vi "UDP Rx Process.vi"(10 "Parameters":variant, 11 "Process":refnum<class "Process.lvclass">) -> ()   [LabVIEW 2019, in "UDP-Custom-Device Engine.lvlib"]
uses:
  UDP-Custom-Device Engine.lvlib
  <vilib>/NI/NIVS Inline Async API/_VS Inline Async API/Process/Process.lvclass
  <vilib>/NI/NIVS Inline Async API/_VS Inline Async API/Process/Process.lvclass/Process.ctl
  <vilib>/NI/NIVS Inline Async API/_VS Inline Async API/Process/Data Member Access/Read Data Access.vi
  <vilib>/NI/NIVS Inline Async API/_VS Inline Async API/Error Handling Process/SubVIs/Error.ConvertArray.vi
  <vilib>/NI/NIVS Inline Async API/_Data Access Engine/Data Access Engine/Data Access Engine.lvclass
  <vilib>/NI VeriStand/VeriStand Data/VeriStand Data.lvlib
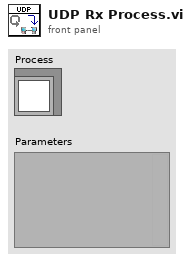
[diagram p1: front panel]
types:
  T1 = typedef "UDP-Custom-Device Engine.lvlib/Engine - Rx Loop Data.ctl" = cluster{"General Resources":T2, "Header Details":T4, "Data Conversion":T6, "Runtime Resources":T8, "New Data Support":T11, "Channel Resources":T13, "Debug Resources":T15}
  T2 = typedef "UDP-Custom-Device Engine.lvlib/Engine - General Resources.ctl" = cluster{"Packet Name":string, "Packet ID":i32, "Local IP Address":string, "Local Port":i32, "Multicast":bool, "Multicast IP Address":u32, "Header Info":bool[], "Byte Order":enum16{"big-endian, network order", "native, host order", "little-endian"}, "Channel Data Types":T3[], "Duplex Packets":refnum<data-value>}
  T3 = typedef "VeriStand Data.lvlib/Typedefs.Data Types.ctl" = enum16{"Boolean", "Single", "Double", "I8", "I16", "I32", "I64", "U8", "U16", "U32", "U64"}
  T4 = typedef "UDP-Custom-Device Shared.lvlib/Shared - Header Details.ctl" = cluster{"Packet Size":u16, "Protocol Revision":u8, "System Definition Version":u64, "Source Node Name":string, "Packet ID":u32, "Number of Channels":u32, "Static Header Size":u16, "Total Header Size":u16, "CustomHeaderLogic":T5}
  T5 = typedef "UDP-Custom-Device Shared.lvlib/Shared - Custom Header.ctl" = cluster{"CustomHeaderON":bool, "CustomHeaderLogic":string}
  T6 = typedef "UDP-Custom-Device Engine.lvlib/Engine - Data Conversion Config.ctl" = cluster{"Byte Buffer":refnum<class "Byte Buffer.lvclass">, "Data Pointers":u64[], "Channel Count":i32, "Mappings":T7[], "Static Header Payload":string, "Packet Count":dbl, "Packet Size":i32}
  T7 = typedef "VeriStand Data.lvlib/Byte Buffer.lvclass/Byte Buffer.Mapping.ctl" = cluster{"pointer":u64, "count":i64, "buffer offset":u64, "data type":T3}
  T8 = typedef "UDP-Custom-Device Engine.lvlib/Engine - Rx Runtime Resources.ctl" = cluster{"Connection ID":refnum<k16>, "Timeout":i32, "ExecutionConfig":T9}
  T9 = typedef "UDP-Custom-Device Engine.lvlib/Engine - Execution Config.ctl" = cluster{"Loop Period":i64, "RT Loop Period":i64, "Untimed Period":u32, "Target Processor":i32, "Priority":i32, "Thread Management":T10}
  T10 = typedef "UDP-Custom-Device Shared.lvlib/Shared - Thread Management.ctl" = enum16{"Untimed (Default)", "Timed (High Priority)"}
  T11 = typedef "UDP-Custom-Device Engine.lvlib/Engine - Rx New Data Options Support.ctl" = cluster{"New Data Option":T12, "Packet Count":dbl}
  T12 = typedef "UDP-Custom-Device Shared.lvlib/Shared - New Data Options.ctl" = enum16{"Timeout Reset", "Counter"}
  T13 = typedef "UDP-Custom-Device Engine.lvlib/Engine - Rx Channel Refs.ctl" = cluster{"Receive Channels":T14, "New Data":T14, "Port":T14}
  T14 = typedef "Data Access Engine.lvlib/Data Access Engine.lvclass/Write.DVR.ctl" = refnum<data-value>
  T15 = typedef "UDP-Custom-Device Engine.lvlib/Engine - Debug Resources.ctl" = cluster{"Debug Mode":bool, "Debug Log File":refnum<file>, "Packet Name":string}
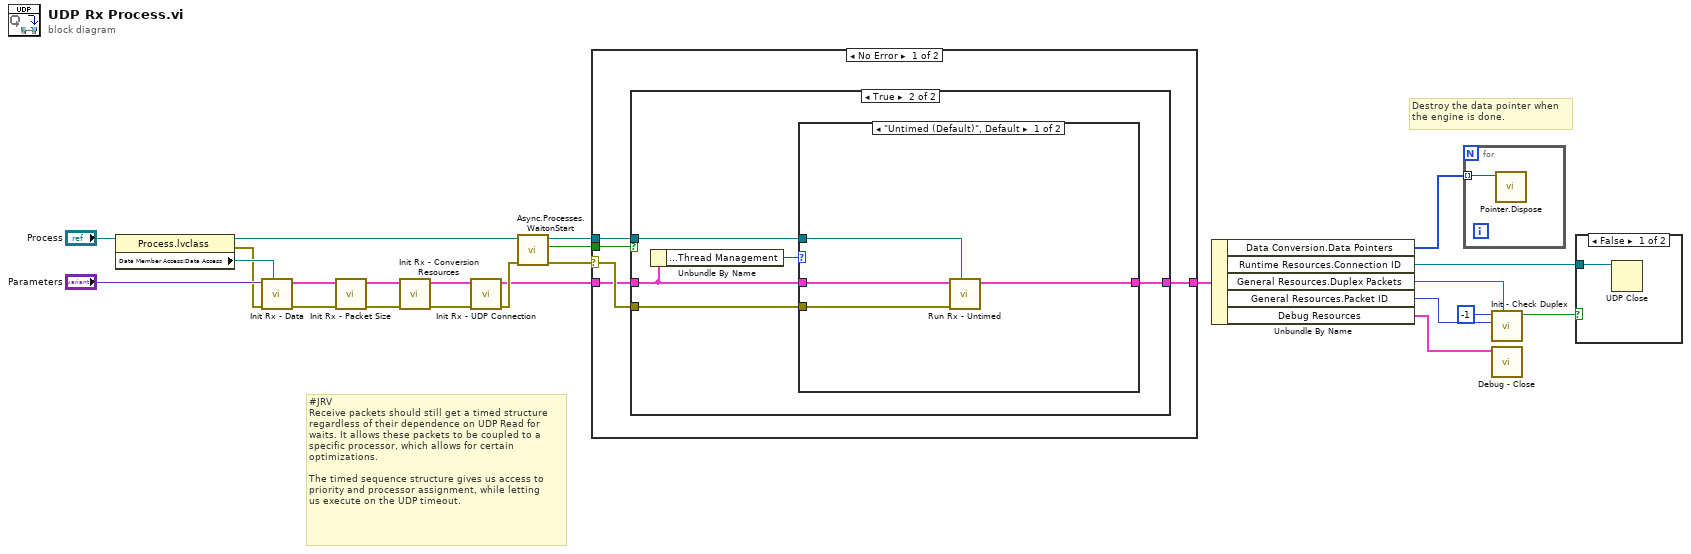
[diagram p0: block diagram]
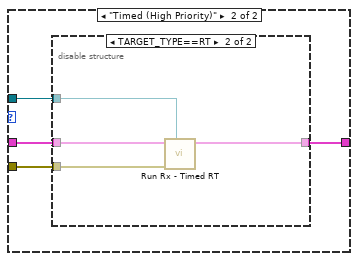
[diagram p3: hidden frame]
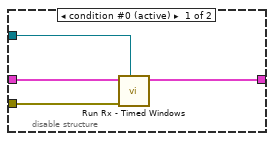
[diagram p4: hidden frame]
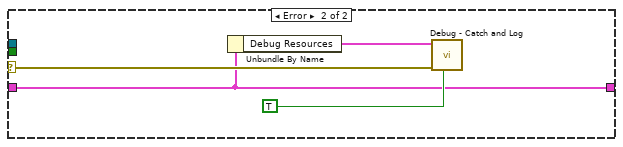
[diagram p5: hidden frame]
diagram:
  # "#JRV\nReceive packets should still get a timed structure\nregardless of their dependence on UDP Read for\nwaits. It allows these packets to be coupled to a\nspecific processor, which allows for certain \noptimizations.\n\nThe timed sequence structure gives us access to\npriority and processor assignment, while letting\nus execute on the UDP timeout."
  # "Destroy the data pointer when\nthe engine is done."
  n1 = property class="Process.lvclass"(reference="Process") -> (reference out=w24:refnum<class "Process.lvclass">, error out=w20:errorcluster, "Data Member Access:Data Access"=w21:refnum<class "Data Access Engine.lvclass">)  [unwired: 1 in]
  n2 = call "Init Rx - Data.vi"("Data Access in"=w21, "error in (no error)"=w20, "Parameters"="Parameters") -> ("error out"=w10:errorcluster, "Rx Loop Data"=w12:T1)  [unwired: 6 in, 1 out]
  n3 = call "Init Rx - Packet Size.vi"("error in (no error)"=w10, "Rx Loop Data"=w12) -> ("error out"=w9:errorcluster, "Rx Loop Data out"=w11:T1)  [unwired: 8 in]
  n4 = call "Init Rx - Conversion Resources.vi"("error in (no error)"=w9, "Rx Loop Data"=w11) -> ("error out"=w13:errorcluster, "Rx Loop Data out"=w14:T1)  [unwired: 8 in]
  n5 = call "Init Rx - UDP Connection.vi"("error in (no error)"=w13, "Rx Loop Data in"=w14) -> ("error out"=w16:errorcluster, "Rx Loop Data out"=w6:T1)  [unwired: 8 in]
  n6 = call <vilib>:"Async.Processes.WaitonStart.vi"("error in (no error)"=w16, "Process"=w24) -> ("error out"=w19:errorcluster, "Execute"=w17:bool, "Process out"=w18:refnum<class "Process.lvclass">)  [unwired: 7 in]
  n7 = case shown="No Error" w19 {
    selector: w19 -> [w27 w53]
    tunnel: w17 -> [w29 _]
    tunnel: w18 -> [w28 _]
    tunnel: w6 -> [w26 w52]
    tunnel: [w25 w52] -> w15
    frame No Error {
      n8 = case shown="True" w29 {
        tunnel: w27 -> [_ w34]
        tunnel: w28 -> [_ w35]
        tunnel: w26 -> [w30 w32]
        tunnel: [w30 w33] -> w25
        frame False {
        }
        frame True {
          n9 = Unbundle By Name(w32) -> ("Runtime Resources.ExecutionConfig.Thread Management"=w31:T10)
          n10 = case shown="\"Untimed (Default)\", Default" w31 {
            tunnel: w35 -> [w36 w43]
            tunnel: w34 -> [w38 w42]
            tunnel: [w37 w41] -> w33
            tunnel: w32 -> [w39 w40]
            frame "Untimed (Default)", Default {
              n11 = call "Run Rx - Untimed.vi"("Process in"=w36, "error in (no error)"=w38, "Rx Loop Data in"=w39) -> ("Rx Loop Data out"=w37:T1)  [unwired: 8 in]
            }
            frame "Timed (High Priority)" {
              n12 = disable-structure shown="TARGET_TYPE==RT" {
                disable-tunnel: w43 -> [w45 w49]
                disable-tunnel: w42 -> [w46 w48]
                disable-tunnel: w40 -> [w47 w51]
                disable-tunnel: [w44 w50] -> w41
                frame condition #0 (active) {
                  n13 = call "Run Rx - Timed Windows.vi"("Process in"=w45, "error in (no error)"=w46, "Rx Loop Data in"=w47) -> ("Rx Loop Data out"=w44:T1)  [unwired: 8 in]
                }
                frame condition #1 {
                  n14 = call "Run Rx - Timed RT.vi"("Process in"=w49, "error in (no error)"=w48, "Rx Loop Data in"=w51) -> ("Rx Loop Data out"=w50:T1)  [unwired: 8 in]
                }
              }
            }
          }
        }
      }
    }
    frame Error {
      n15 = Unbundle By Name(w52) -> ("Debug Resources"=w54:T15)
      n16 = call "Debug - Catch and Log.vi"("Clear Error?"=TRUE, "error in (no error)"=w53, "Debug Resources"=w54) -> ()  [unwired: 8 in, 1 out]
    }
  }
  n17 = Unbundle By Name(w15) -> ("Data Conversion.Data Pointers"=w8:u64[], "Runtime Resources.Connection ID"=w7:refnum<k16>, "General Resources.Duplex Packets"=w2:refnum<data-value>, "General Resources.Packet ID"=w4:i32, "Debug Resources"=w1:T15)
  n18 = for {
    tunnel: w8 -> [w56] mode=indexing
    n19 = call <vilib>:"Pointer.Dispose.vi"("pointer"=w56) -> ()  [unwired: 9 in, 2 out]
  }
  n20 = call "Init - Check Duplex.vi"("Duplex Packets"=w2, "Receive Packet ID"=w4, "Transmit Packet ID"=-1 ("Receive Packet ID")) -> ("Is Duplex?"=w3:bool)  [unwired: 6 in, 2 out]
  n21 = call "Debug - Close.vi"("Debug Resources"=w1) -> ()  [unwired: 10 in, 1 out]
  n22 = case shown="False" w3 {
    tunnel: w7 -> [w57 _]
    frame False {
      n23 = UDP Close(connection ID=w57) -> ()  [unwired: 1 in, 2 out]
    }
    frame True {
    }
  }
